vi "生成word报表.vi"(0 "Array输入":refnum<vi>, 1 "产品序号":string, 2 "标注图":T1(plugin-control), 4 "测试人":string, 5 "部位":string, 6 "类型":string, 7 "产品序号":string, 8 "原图":T1(plugin-control) caption="Original Image") -> (14 "报告生成路径":path)   [LabVIEW 2018]
uses:
  <vilib>/Utility/NIReport.llb/Report Type.ctl
  <vilib>/Utility/NIReport.llb/Append Report Text (str wrap).vi
  <vilib>/addons/_office/word.llb/Word Edit Cell ([dbl]).vi
  <vilib>/addons/_office/word.llb/Word Edit Cell (str).vi
  <vilib>/Utility/NIReport.llb/Append Image to Report (path wrap).vi
  <vilib>/Utility/NIReport.llb/NI_report.lvclass
  <vilib>/addons/_office/NI_ReportGenerationToolkit.lvlib
  <vilib>/Utility/NIReport.llb/Word/NI_Word.lvclass
  <vilib>/Utility/NIReport.llb/NI_ReportGenerationCore.lvlib
panel:
  out "累计缺陷占比":dbl
  out "值":dbl[][](array[numeric])
  out "Z值":dbl[](array[numeric])
  out "缺陷个数":i32
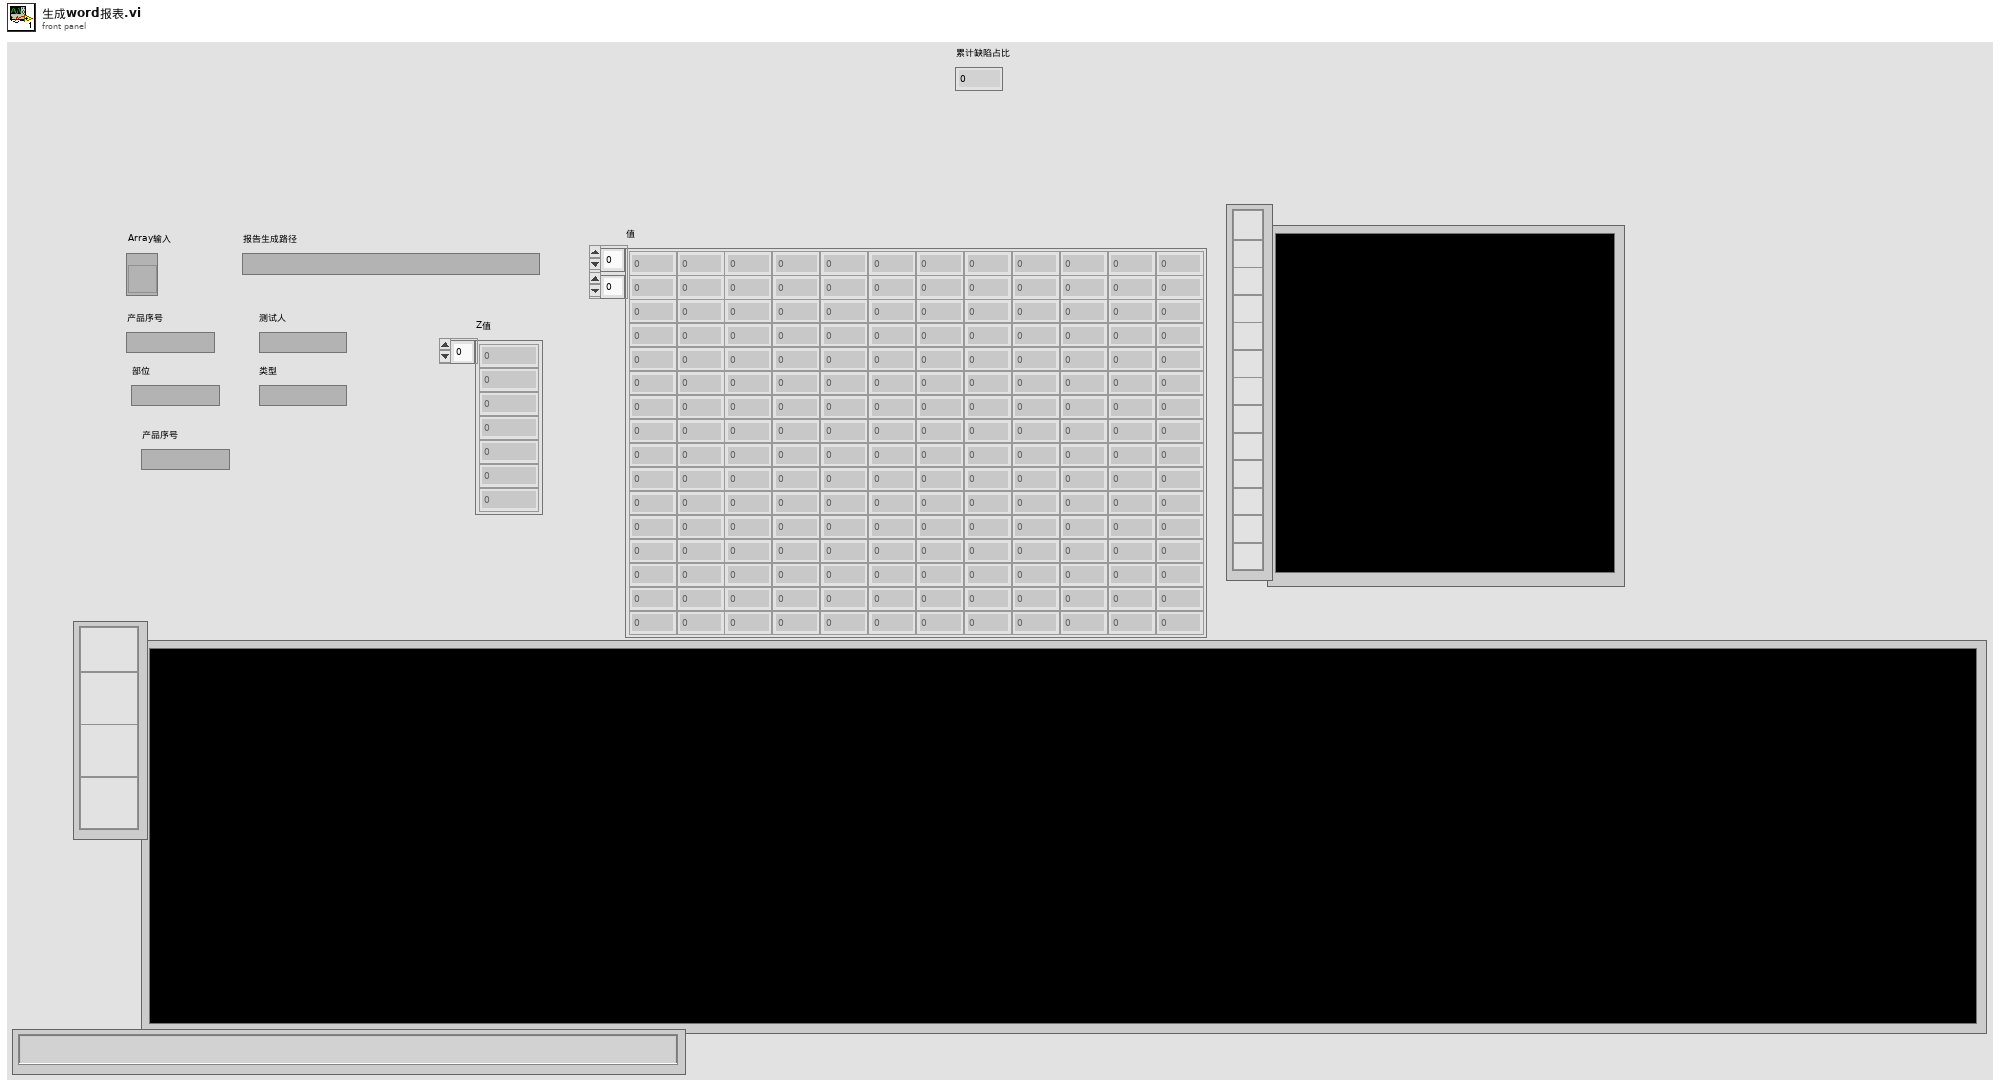
[diagram p1: front panel]
types:
  T1 = typedef "IMAQ Image.ctl" = refnum<image>
  T2 = cluster{"position (Excel)":cluster{"row":i32, "column":i32}, "name (Excel)":string, "bookmark (Word)":string}
  T3 = typedef "NI_ReportGenerationCore.lvlib/Report Type.ctl" = enum16{"HTML", "Word", "Excel"}
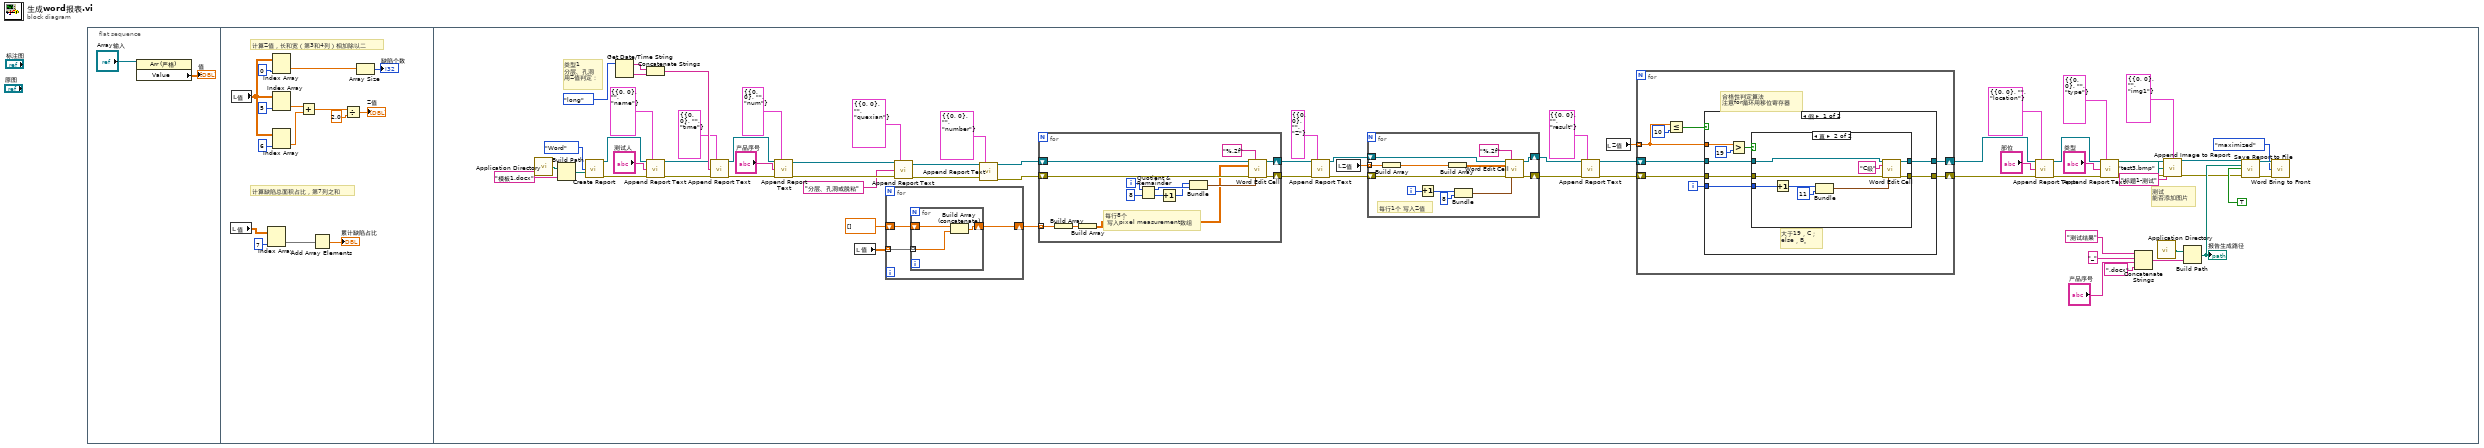
[diagram p0: block diagram]
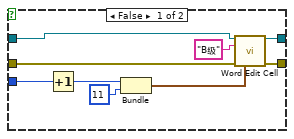
[diagram p2: hidden frame]
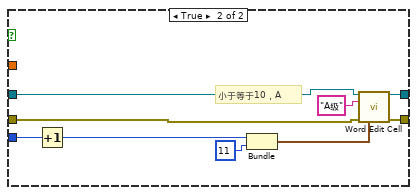
[diagram p3: hidden frame]
diagram:
  n1 = flat-sequence {
    frame #0 {
      n2 = property class="Arr (严格)"(reference="Array输入") -> ("Value"=→"值":dbl[][])  [unwired: 1 in, 2 out]
    }
    frame #1 {
      # "计算缺陷总面积占比，第7列之和"
      # "计算Z值，长和宽（第3和4列）相加除以二"
      n3 = local read "值"() -> (w6:dbl[][])
      n4 = local read "值"() -> (w17:dbl[][])
      n5 = Index Array(array=w6, index (col)=7 ("禁用的索引 (列)")) -> (element=w4:dbl[])  [unwired: 1 in]
      n6 = Index Array(array=w17, index (col)=0 ("禁用的索引 (列)")) -> (element=w14:dbl[])  [unwired: 1 in]
      n7 = Index Array(array=w17, index (col)=5 ("索引")) -> (element=w11:dbl[])  [unwired: 1 in]
      n8 = Index Array(array=w17, index (col)=6 ("索引")) -> (element=w12:dbl[])  [unwired: 1 in]
      n9 = Add(x=w11, y=w12) -> (x+y=w13:dbl[])
      n10 = Add Array Elements(numeric array=w4) -> (sum=→"累计缺陷占比":dbl)
      n11 = Divide(x=w13, y=2.0) -> (x/y=→"Z值":dbl[])
      n12 = Array Size(array=w14) -> (size(s)=→"缺陷个数":i32)
    }
    frame #2 {
      # "测试\n能否添加图片"
      # "类型1\n分层、孔洞\n用Z值判定："
      n13 = call <vilib>:"Application Directory.vi"() -> ("Application Directory"=w63:path)
      n14 = Build Path(base path=w63, name or relative path="模板1.docx") -> (appended path=w62:path)
      n15 = call <vilib>:"Create Report.vi"("report type"=Report_Type."Word" ("Report Type"), "template (empty)"=w62) -> ("report out"=w55:refnum<class "NI_report.lvclass">, "error out"=w52:errorcluster)  [unwired: 12 in]
      n16 = Get Date/Time String(date format (0)=enum16{"short", "long", "abbreviated"}."long" ("日期格式(0)")) -> (date string=w61:string, time string=w59:string)  [unwired: 2 in]
      n17 = Concatenate Strings(w61, w59) -> (w60:string)
      n18 = call-poly <vilib>:"Append Report Text.vi"("report in"=w55, "MS Office parameters"=T2 {"position (Excel)"={"row"=0, "column"=0}, "name (Excel)"="", "bookmark (Word)"="name"}, "text"="测试人", "error in (no error)"=w52) -> ("report out"=w54:refnum<class "NI_report.lvclass">, "error out"=w53:errorcluster)  [unwired: 8 in, 2 out]
      n19 = call-poly <vilib>:"Append Report Text.vi"("report in"=w54, "MS Office parameters"=T2 {"position (Excel)"={"row"=0, "column"=0}, "name (Excel)"="", "bookmark (Word)"="time"}, "text"=w60, "error in (no error)"=w53) -> ("report out"=w58:refnum<class "NI_report.lvclass">, "error out"=w57:errorcluster)  [unwired: 8 in, 2 out]
      n20 = call-poly <vilib>:"Append Report Text.vi"("report in"=w58, "MS Office parameters"=T2 {"position (Excel)"={"row"=0, "column"=0}, "name (Excel)"="", "bookmark (Word)"="num"}, "text"="产品序号", "error in (no error)"=w57) -> ("report out"=w27:refnum<class "NI_report.lvclass">, "error out"=w26:errorcluster)  [unwired: 8 in, 2 out]
      n21 = local read "值"() -> (w67:dbl[][])
      n22 = for {
        tunnel: w67 -> [w144] mode=indexing
        shift-right: [w142] -> w56
        shift-left: dbl[] [] ("元素") -> [w143]
        n23 = for {
          tunnel: w144 -> [w147] mode=indexing
          shift-right: [w145] -> w142
          shift-left: w143 -> [w146]
          n24 = Build Array (concatenate)(w146, w147) -> (w145:dbl[])
        }
      }
      n25 = call-poly <vilib>:"Append Report Text.vi"("report in"=w27, "MS Office parameters"=T2 {"position (Excel)"={"row"=0, "column"=0}, "name (Excel)"="", "bookmark (Word)"="quexian"}, "text"="分层、孔洞或脱粘", "error in (no error)"=w26) -> ("report out"=w29:refnum<class "NI_report.lvclass">, "error out"=w28:errorcluster)  [unwired: 8 in, 2 out]
      n26 = call-poly <vilib>:"Append Report Text.vi"("report in"=w29, "MS Office parameters"=T2 {"position (Excel)"={"row"=0, "column"=0}, "name (Excel)"="", "bookmark (Word)"="number"}, "error in (no error)"=w28) -> ("report out"=w65:refnum<class "NI_report.lvclass">, "error out"=w64:errorcluster)  [unwired: 9 in, 2 out]
      n27 = for {
        shift-right: [w161] -> w48
        shift-left: w65 -> [w156]
        shift-right: [w160] -> w86
        shift-left: w64 -> [w155]
        tunnel: w56 -> [w149] mode=indexing
        i -> [w157]
        # "每行8个\n 写入pixel measurement数组"
        n28 = Build Array(w149) -> (w151:dbl[])
        n29 = Build Array(w151) -> (w150:dbl[][])
        n30 = Quotient & Remainder(x=w157, y=8) -> (x-y*floor(x/y)=w154:i32, floor(x/y)=w153:i32)
        n31 = Increment(x=w153) -> (x+1=w152:i32)
        n32 = Bundle(w152, w154) -> (w159:cluster{i32, i32})  [unwired: 1 in]
        n33 = call-poly <vilib>:"Word Edit Cell.vi"("report in"=w156, "format string (%.3f)"="%.2f", "value"=w150, "error in (no error)"=w155, "start (0, 0)"=w159) -> ("report out"=w161:refnum<class "NI_report.lvclass">, "error out"=w160:errorcluster)  [unwired: 9 in]
      }
      n34 = call-poly <vilib>:"Append Report Text.vi"("report in"=w48, "MS Office parameters"=T2 {"position (Excel)"={"row"=0, "column"=0}, "name (Excel)"="", "bookmark (Word)"="Z"}, "error in (no error)"=w86) -> ("report out"=w75:refnum<class "NI_report.lvclass">, "error out"=w74:errorcluster)  [unwired: 9 in, 2 out]
      n35 = local read "Z值"() -> (w68:dbl[])
      n36 = for {
        shift-right: [w141] -> w71
        shift-left: w75 -> [w138]
        shift-right: [w140] -> w70
        shift-left: w74 -> [w137]
        tunnel: w68 -> [w133] mode=indexing
        i -> [w131]
        # "每行1个 写入Z值"
        n37 = Build Array(w133) -> (w135:dbl[])
        n38 = Increment(x=w131) -> (x+1=w136:i32)
        n39 = Build Array(w135) -> (w134:dbl[][])
        n40 = Bundle(w136, "y"=8) -> (w139:cluster{i32, "y":i32})  [unwired: 1 in]
        n41 = call-poly <vilib>:"Word Edit Cell.vi"("report in"=w138, "format string (%.3f)"="%.2f", "value"=w134, "error in (no error)"=w137, "start (0, 0)"=w139) -> ("report out"=w141:refnum<class "NI_report.lvclass">, "error out"=w140:errorcluster)  [unwired: 9 in]
      }
      n42 = call-poly <vilib>:"Append Report Text.vi"("report in"=w71, "MS Office parameters"=T2 {"position (Excel)"={"row"=0, "column"=0}, "name (Excel)"="", "bookmark (Word)"="result"}, "error in (no error)"=w70) -> ("report out"=w72:refnum<class "NI_report.lvclass">, "error out"=w73:errorcluster)  [unwired: 9 in, 2 out]
      n43 = local read "Z值"() -> (w69:dbl[])
      n44 = for {
        shift-right: [w88] -> w49
        shift-left: w72 -> [w91]
        shift-right: [w89] -> w50
        shift-left: w73 -> [w90]
        tunnel: w69 -> [w87] mode=indexing
        i -> [w92]
        # "合格性判定算法\n注意for循环用移位寄存器"
        n45 = Less Or Equal?(x=w87, y=10) -> (x <= y?=w93:bool)
        n46 = case shown="假" w93 {
          tunnel: w92 -> [w99 w127]
          tunnel: w91 -> [w98 w126]
          tunnel: w90 -> [w97 w125]
          tunnel: [w95 w124] -> w89
          tunnel: [w96 w123] -> w88
          tunnel: w87 -> [w102 _]
          frame False {
            # "大于19，C；\nelse，B。"
            n47 = Greater?(x=w102, y=19) -> (0:w100:bool)
            n48 = case shown="真" w100 {
              tunnel: w99 -> [w103 w116]
              tunnel: w98 -> [w107 w115]
              tunnel: w97 -> [w106 w114]
              tunnel: [w105 w113] -> w96
              tunnel: [w104 w112] -> w95
              frame False {
                n49 = Increment(x=w103) -> (x+1=w111:i32)
                n50 = Bundle(w111, "y"=11) -> (w110:cluster{i32, "y":i32})  [unwired: 1 in]
                n51 = call-poly <vilib>:"Word Edit Cell.vi"("report in"=w107, "value"="B级", "error in (no error)"=w106, "start (0, 0)"=w110) -> ("report out"=w105:refnum<class "NI_report.lvclass">, "error out"=w104:errorcluster)  [unwired: 10 in]
              }
              frame True {
                n52 = Increment(x=w116) -> (x+1=w120:i32)
                n53 = Bundle(w120, "y"=11) -> (w119:cluster{i32, "y":i32})  [unwired: 1 in]
                n54 = call-poly <vilib>:"Word Edit Cell.vi"("report in"=w115, "value"="C级", "error in (no error)"=w114, "start (0, 0)"=w119) -> ("report out"=w113:refnum<class "NI_report.lvclass">, "error out"=w112:errorcluster)  [unwired: 10 in]
              }
            }
          }
          frame True {
            # "小于等于10，A"
            n55 = Increment(x=w127) -> (x+1=w129:i32)
            n56 = Bundle(w129, "y"=11) -> (w121:cluster{i32, "y":i32})  [unwired: 1 in]
            n57 = call-poly <vilib>:"Word Edit Cell.vi"("report in"=w126, "value"="A级", "error in (no error)"=w125, "start (0, 0)"=w121) -> ("report out"=w123:refnum<class "NI_report.lvclass">, "error out"=w124:errorcluster)  [unwired: 10 in]
          }
        }
      }
      n58 = call-poly <vilib>:"Append Report Text.vi"("report in"=w49, "MS Office parameters"=T2 {"position (Excel)"={"row"=0, "column"=0}, "name (Excel)"="", "bookmark (Word)"="location"}, "text"="部位", "error in (no error)"=w50) -> ("report out"=w83:refnum<class "NI_report.lvclass">, "error out"=w82:errorcluster)  [unwired: 8 in, 2 out]
      n59 = call-poly <vilib>:"Append Report Text.vi"("report in"=w83, "MS Office parameters"=T2 {"position (Excel)"={"row"=0, "column"=0}, "name (Excel)"="", "bookmark (Word)"="type"}, "text"="类型", "error in (no error)"=w82) -> ("report out"=w24:refnum<class "NI_report.lvclass">, "error out"=w21:errorcluster)  [unwired: 8 in, 2 out]
      n60 = Concatenate Strings("测试结果" ("字符串"), "_" ("名称或相对路径"), "产品序号", ".docx" ("名称或相对路径")) -> (w79:string)
      n61 = call <vilib>:"Application Directory.vi"() -> ("Application Directory"=w80:path)
      n62 = call-poly <vilib>:"Append Image to Report.vi"("report in"=w24, "MS Office parameters"=T2 {"position (Excel)"={"row"=0, "column"=0}, "name (Excel)"="", "bookmark (Word)"="img1"}, "path or URL of image"=path "test3.bmp", "caption or alternative string"="标题1-测试", "error in (no error)"=w21) -> ("report out"=w23:refnum<class "NI_report.lvclass">, "error out"=w22:errorcluster)  [unwired: 7 in, 2 out]
      n63 = Build Path(base path=w80, name or relative path=w79) -> (appended path=w81:path)
      "报告生成路径" <- w81
      n64 = call-dynamic "Save Report to File.vi"("report in"=w23, "report file path"=w81, "prompt to replace? (F)"=TRUE, "error in (no error)"=w22) -> ("report out"=w78:refnum<class "NI_report.lvclass">, "error out"=w77:errorcluster)  [unwired: 10 in]
      n65 = call <vilib>:"Word Bring to Front.vi"("report in"=w78, "window state (maximized)"=enum16{"maximized", "minimized", "normal"}."maximized", "error in (no error)"=w77) -> ()  [unwired: 11 in, 2 out]
    }
  }
